vi "sandify_test.vi"() -> ()   [LabVIEW 2020]
panel:
  out "Numeric 2":sgl
  out "Numeric":sgl
  out "output variable 2":sgl
  out "output variable":sgl
  in  "XY Input":cluster{"X":dbl, "Y":dbl}
  out "XY":cluster{"X":dbl, "Y":dbl}
  in  "Stop":bool
  out "XY Graph":cluster{dbl[], dbl[]}(graph)
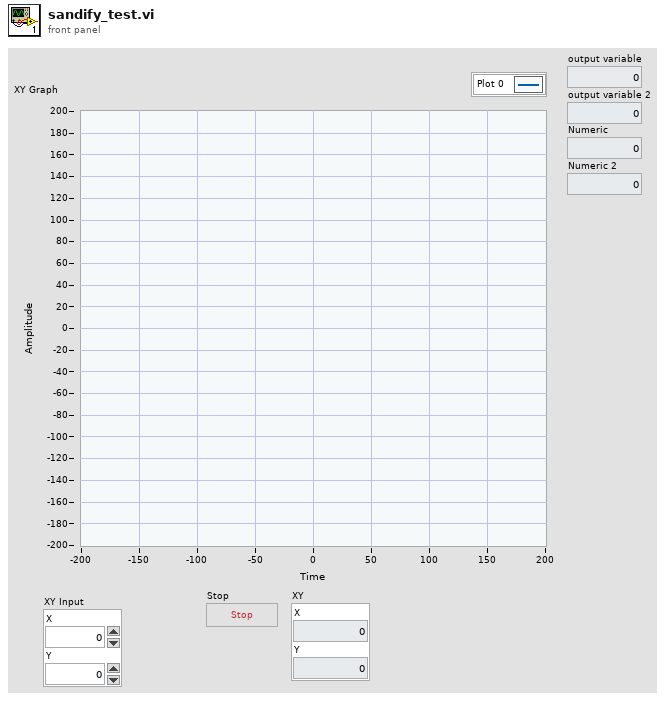
[diagram p1: front panel]
types:
  T1 = typedef "LVPoint32TypeDef.ctl" = cluster{"Horizontal":i32, "Vertical":i32}
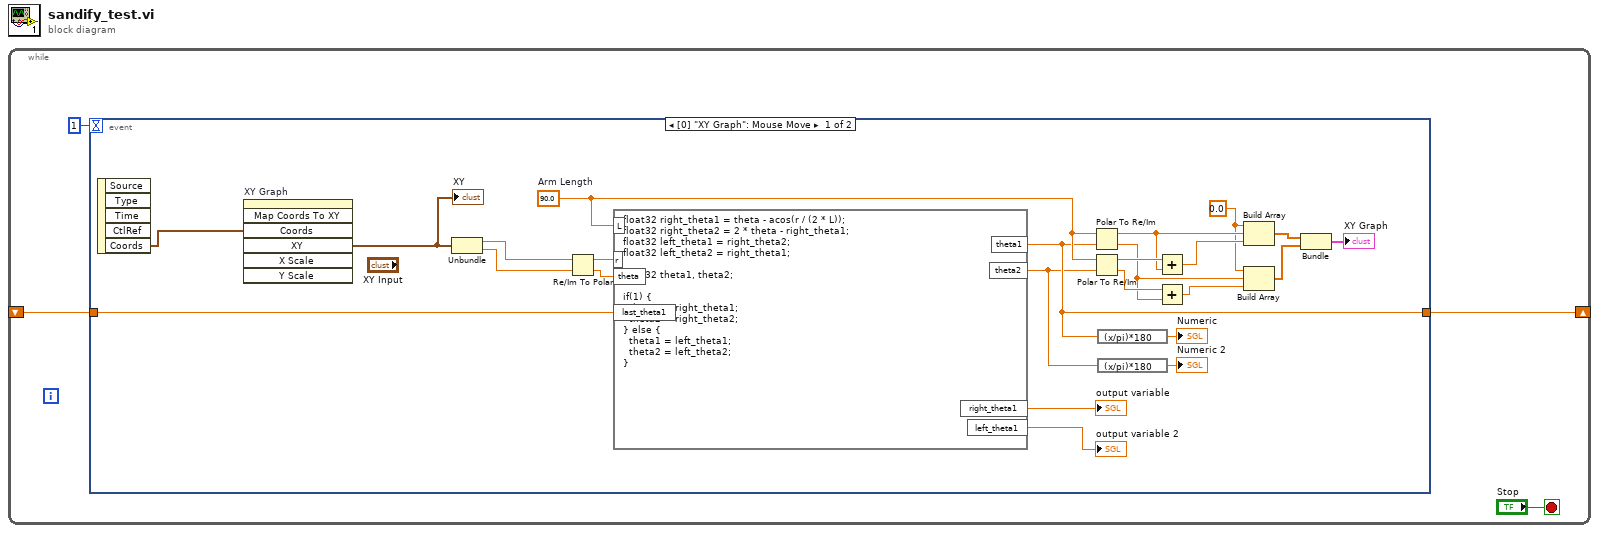
[diagram p0: block diagram]
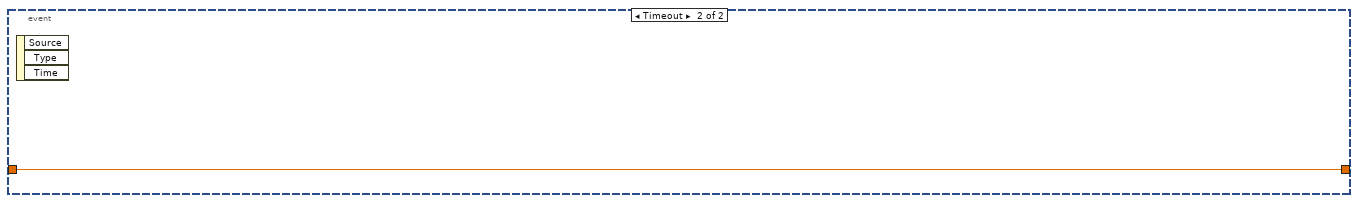
[diagram p2: hidden frame]
diagram:
  n1 = while {
    shift-right: [w3] -> _
    shift-left: _ -> [w2]
    stop <- "Stop" stop-if-true
    n2 = event shown="[0] \"XY Graph\": Mouse Move" {
      selector: _ -> [_ _]
      dyn-events: _ -> [_ _]
      timeout: 1 -> [_ _]
      tunnel: [w9 w29] -> w3
      tunnel: w2 -> [w15 w29]
      event "XY Graph": Mouse Move {
        w16 = 0.0 ("element")
        w26 = 90.0  # Arm Length
        n3 = event-data() -> ("Coords"=w12:T1)  [unwired: 1 in, 4 out]
        n4 = invoke on="XY Graph" class="XYGraph (strict)" method="Map Coords To XY"("Coords"=w12) -> ("XY"=w5:cluster{"X":dbl, "Y":dbl})  [unwired: 6 in, 6 out]
        "XY" <- w5
        n5 = Unbundle(w5) -> ("X"=w14:dbl, "Y"=w13:dbl)
        n6 = Re/Im To Polar(2:w13, 3:w14) -> (0:w27:dbl, 1:w28:dbl)
        n7 = formula code="float32 right_theta1 = theta - acos(r / (2 * L));\nfloat32 right_theta2 = 2 * theta - right_theta1;\nfloat32 left_theta1 = right_theta2;\nfloat32 left_theta2 = right_theta1;\n\nfloat32 theta1, theta2;\n\nif(1) {\n  theta1 = right_theta1;\n  theta2 = right_theta2;\n} else {\n  theta1 = left_theta1;\n  theta2 = left_theta2;\n}"("r"=w28, "theta"=w27, "L"=w26, "last_theta1"=w15) -> ("theta1"=w9:sgl, "theta2"=w8:sgl, "right_theta1"=→"output variable":sgl, "left_theta1"=→"output variable 2":sgl)
        n8 = Polar To Re/Im(2:w9, 3:w26) -> (0:w21:dbl, 1:w23:dbl)
        n9 = Polar To Re/Im(2:w8, 3:w26) -> (0:w24:dbl, 1:w25:dbl)
        n10 = expression code="(x/pi)*180"(w9) -> (→"Numeric":sgl)
        n11 = expression code="(x/pi)*180"(w8) -> (→"Numeric 2":sgl)
        n12 = Add(x=w25, y=w23) -> (x+y=w22:dbl)
        n13 = Add(x=w24, y=w21) -> (x+y=w20:dbl)
        n14 = Build Array(w16, w23, w22) -> (w19:dbl[])
        n15 = Build Array(w16, w21, w20) -> (w18:dbl[])
        n16 = Bundle(w19, w18) -> (→"XY Graph":cluster{dbl[], dbl[]})  [unwired: 1 in]
      }
      event Timeout {
        n17 = event-data() -> ()  [unwired: 1 in, 3 out]
      }
    }
  }
